vi "Extract the same Property Channels.vi"(8 "error in (no error)":errorcluster, 10 "Property Name":string="pkid", 11 "Channel Refs in":T1[](array[typedef]) format="%.0x") -> (0 "error out":errorcluster, 1 "Property Value":u8, 2 "Extracted the same pkid Channel Refs":T1[](array[typedef]) format="%.0x", 3 "Channel Refs Remaining":T1[](array[typedef]) format="%.0x")   [LabVIEW 2023, in "Vires VTD System Explorer.lvlib"]
uses:
  Vires VTD System Explorer.lvlib
  <vilib>/NI VeriStand/Custom Device API/Custom Device Item Ref.ctl
  <vilib>/NI VeriStand/Custom Device API/Get Item Property (Variant).vi
  <vilib>/NI VeriStand/Custom Device API/Custom Device API.lvlib
panel:
  out "Check?":bool
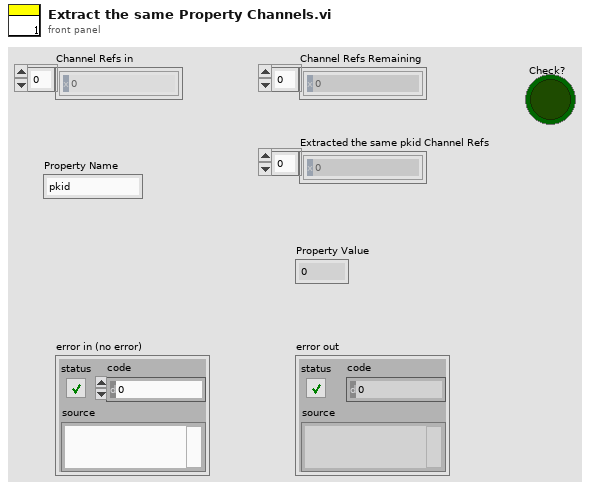
[diagram p1: front panel]
types:
  T1 = typedef "Custom Device API.lvlib/Custom Device Item Ref.ctl" = u64
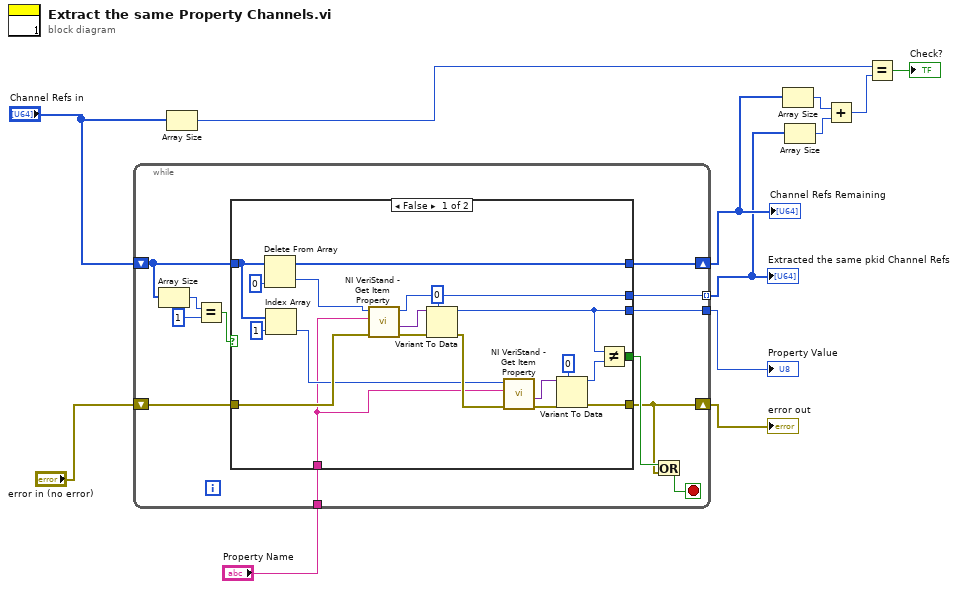
[diagram p0: block diagram]
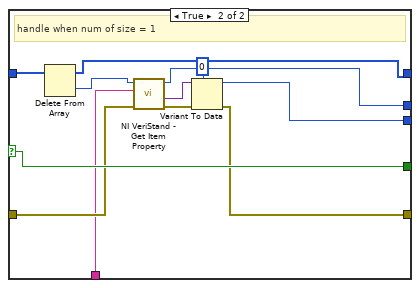
[diagram p2: hidden frame]
diagram:
  n1 = while {
    shift-right: [w15] -> w10
    shift-left: "error in (no error)" -> [w24]
    tunnel: [w23] -> w7 mode=indexing
    tunnel: [w22] -> w12
    shift-right: [w21] -> w8
    shift-left: "Channel Refs in" -> [w20]
    tunnel: "Property Name" -> [w13]
    stop <- w14 stop-if-true
    n2 = Array Size(array=w20) -> (size(s)=w19:i32)
    n3 = Equal?(x=w19, y=1) -> (x = y?=w17:bool)
    n4 = case shown="False" w17 {
      selector: w17 -> [_ w56]
      tunnel: [w39 w50] -> w15
      tunnel: w24 -> [w38 w51]
      tunnel: [w34 w56] -> w16
      tunnel: [w33 w48] -> w23
      tunnel: [w32 w49] -> w22
      tunnel: [w28 w46] -> w21
      tunnel: w20 -> [w26 w47]
      tunnel: w13 -> [w25 w45]
      frame False {
        n5 = Delete From Array(array=w26, index=0) -> (deleted portion=w29:T1, array with subset deleted=w28:T1[])  [unwired: 1 in]
        n6 = Index Array(array=w26, index=1) -> (element=w27:T1)
        n7 = call-poly <vilib>:"NI VeriStand - Get Item Property.vi"("error in (no error)"=w38, "Property Name"=w25, "Item Ref in"=w29) -> ("error out"=w44:errorcluster, "Value"=w43:variant, "Item Ref out"=w33:T1)  [unwired: 5 in, 1 out]
        n8 = Variant To Data(error in=w44, type=u8 0, Variant=w43) -> (data=w32:u8, error out=w42:errorcluster)
        n9 = call-poly <vilib>:"NI VeriStand - Get Item Property.vi"("error in (no error)"=w42, "Property Name"=w25, "Item Ref in"=w27) -> ("error out"=w41:errorcluster, "Value"=w40:variant)  [unwired: 5 in, 2 out]
        n10 = Variant To Data(error in=w41, type=u8 0, Variant=w40) -> (data=w36:u8, error out=w39:errorcluster)
        n11 = Not Equal?(x=w32, y=w36) -> (x != y?=w34:bool)
      }
      frame True {
        # "handle when num of size = 1"
        n12 = Delete From Array(array=w47) -> (deleted portion=w52:T1, array with subset deleted=w46:T1[])  [unwired: 2 in]
        n13 = call-poly <vilib>:"NI VeriStand - Get Item Property.vi"("error in (no error)"=w51, "Property Name"=w45, "Item Ref in"=w52) -> ("error out"=w55:errorcluster, "Value"=w54:variant, "Item Ref out"=w48:T1)  [unwired: 5 in, 1 out]
        n14 = Variant To Data(error in=w55, type=u8 0, Variant=w54) -> (data=w49:u8, error out=w50:errorcluster)
      }
    }
    n15 = Or(x=w16, y=w15) -> (x .or. y?=w14:bool)
  }
  "Property Value" <- w12
  "Channel Refs Remaining" <- w8
  "Extracted the same pkid Channel Refs" <- w7
  "error out" <- w10
  n16 = Array Size(array="Channel Refs in") -> (size(s)=w6:i32)
  n17 = Array Size(array=w8) -> (size(s)=w5:i32)
  n18 = Array Size(array=w7) -> (size(s)=w4:i32)
  n19 = Add(x=w5, y=w4) -> (x+y=w3:i32)
  n20 = Equal?(x=w6, y=w3) -> (x = y?=→"Check?":bool)
